vi "Wind Turbine Set Turbine Speed.vi"(0 "Data Refnum":T1, 7 "Turbine Speed (RPM)":dbl, 11 "error in (no error)":errorcluster) -> (4 "Data Refnum out":T1, 15 "error out":errorcluster)   [LabVIEW 2011, in "SEQ - Solution.lvlib"]
doc: "One VI in the solution for the Wind Turbine class. This group of VIs is built on the SEQ design pattern and illustrates the power of references and named queues.\n\nAAL 9/09"
uses:
  SEQ - Solution.lvlib
  Controls/Wind Turbine DataRef.ctl
  Controls/Wind Turbine Data.ctl
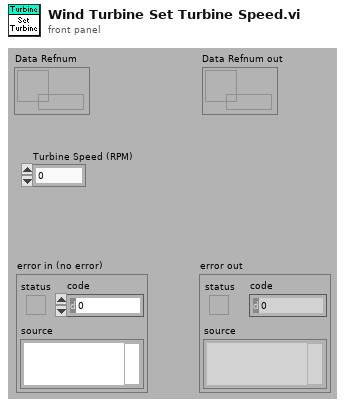
[diagram p1: front panel]
types:
  T1 = typedef "SEQ - Solution.lvlib/Wind Turbine DataRef.ctl" = refnum<queue>
  T2 = typedef "SEQ - Solution.lvlib/Wind Turbine Data.ctl" = cluster{" Wind Speed (ms)":dbl, "Turbine Speed (RPM)":dbl, "Angle Attack (Degs.)":dbl, "Current Power (kW)":dbl, "Energy Generation (kW*hr)":dbl}
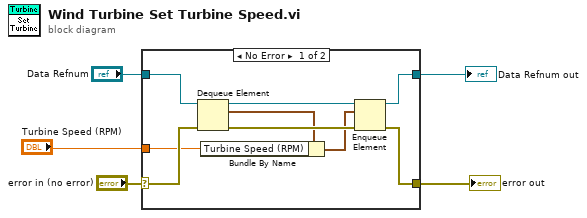
[diagram p0: block diagram]
diagram:
  n1 = case shown="No Error" "error in (no error)" {
    selector: "error in (no error)" -> [w11 w16]
    tunnel: [w10 w16] -> w4
    tunnel: "Data Refnum" -> [w12 w15]
    tunnel: [w9 w15] -> w3
    tunnel: "Turbine Speed (RPM)" -> [w6 _]
    frame No Error {
      n2 = Dequeue Element(queue=w12, error in (no error)=w11) -> (queue out=w14:T1, element=w8:T2, error out=w13:errorcluster)  [unwired: 1 in, 1 out]
      n3 = Bundle By Name(cluster=w8, "Turbine Speed (RPM)"=w6) -> (w7:T2)
      n4 = Enqueue Element(queue=w14, element=w7, error in (no error)=w13) -> (queue out=w9:T1, error out=w10:errorcluster)  [unwired: 1 in, 1 out]
    }
    frame Error {
    }
  }
  "error out" <- w4
  "Data Refnum out" <- w3
